vi "MeasureRMS.vi"(10 "Parameters":T1={"Sampling Rate (Hz)"=100000.0, "# of Samples"=1000.0}) -> (1 "RMS":dbl, 2 "Waveform Graph":dynamicdata(graph))   [LabVIEW 2014]
uses:
  <vilib>/Analysis/NI_AALPro.lvlib
panel:
  out "error out":errorcluster
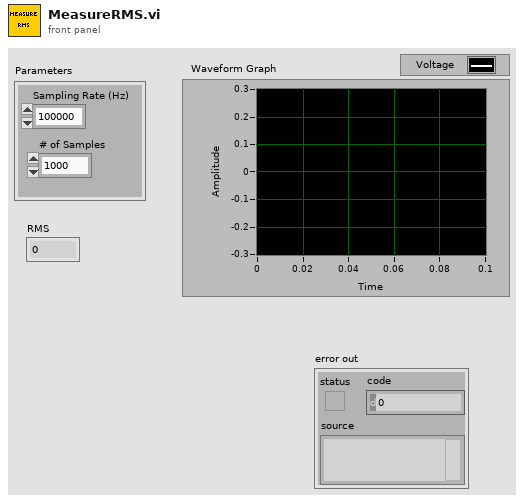
[diagram p1: front panel]
types:
  T1 = cluster{"Sampling Rate (Hz)":dbl, "# of Samples":dbl}
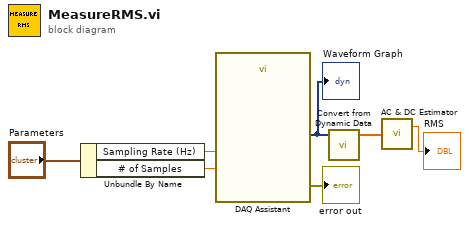
[diagram p0: block diagram]
diagram:
  n1 = Unbundle By Name("Parameters") -> ("Sampling Rate (Hz)"=w2:dbl, "# of Samples"=w1:dbl)
  n2 = call "DAQ Assistant"("rate"=w2, "number of samples"=w1) -> ("data"=w7:dynamicdata, "error out"=→"error out":errorcluster)  [unwired: 15 in, 1 out]
  "Waveform Graph" <- w7
  n3 = call "Convert from Dynamic Data"("Dynamic Data Type"=w7) -> ("Array"=w6:dbl[])  [unwired: 3 in]
  n4 = call <vilib>:"AC & DC Estimator.vi"("Signal (V)"=w6) -> ("AC estimate (Vrms)"=→"RMS":dbl)  [unwired: 1 out]
